vi "Compute Gamma.vi"(10 "Beta":dbl[][](array[numeric]), 11 "Alpha":dbl[][](array[numeric])) -> (3 "Gamma":dbl[][](array[numeric]))   [LabVIEW 2014, in "HMM.lvlib"]
doc: "Calculates the value of gamma."
uses:
  HMM.lvlib
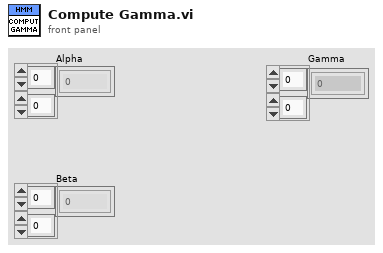
[diagram p1: front panel]
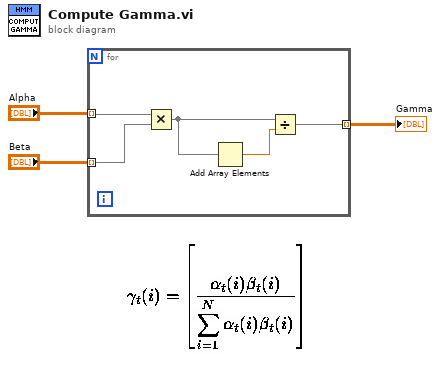
[diagram p0: block diagram]
diagram:
  n1 = for {
    tunnel: "Alpha" -> [w8] mode=indexing
    tunnel: "Beta" -> [w7] mode=indexing
    tunnel: [w4] -> w3 mode=indexing
    n2 = Multiply(x=w8, y=w7) -> (x*y=w6:dbl[])
    n3 = Add Array Elements(numeric array=w6) -> (sum=w5:dbl)
    n4 = Divide(x=w6, y=w5) -> (x/y=w4:dbl[])
  }
  "Gamma" <- w3
